vi "json_object.vi"(5 "text":string, 7 "ch":string, 9 "at":i32, 11 "error in (no error)":errorcluster) -> (4 "object":variant, 6 "text dup":string, 8 "ch out":string, 10 "at out":i32, 15 "error out":errorcluster)   [LabVIEW 2011]
doc: "Recursively return a JSON object (anything wrapped with {})."
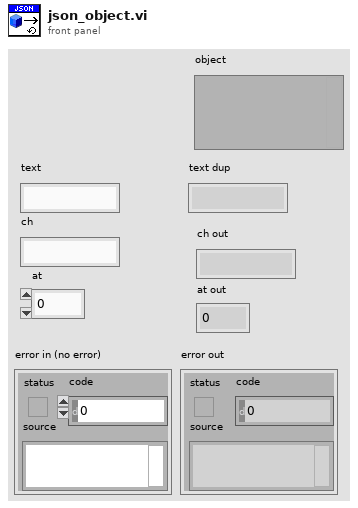
[diagram p1: front panel]
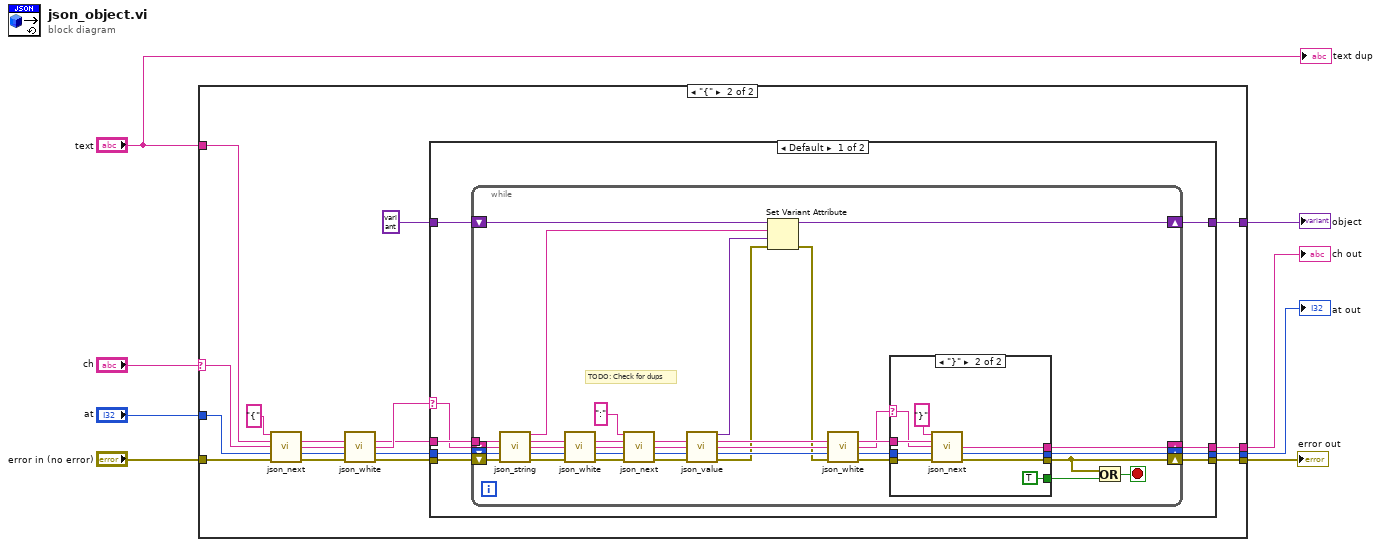
[diagram p0: block diagram]
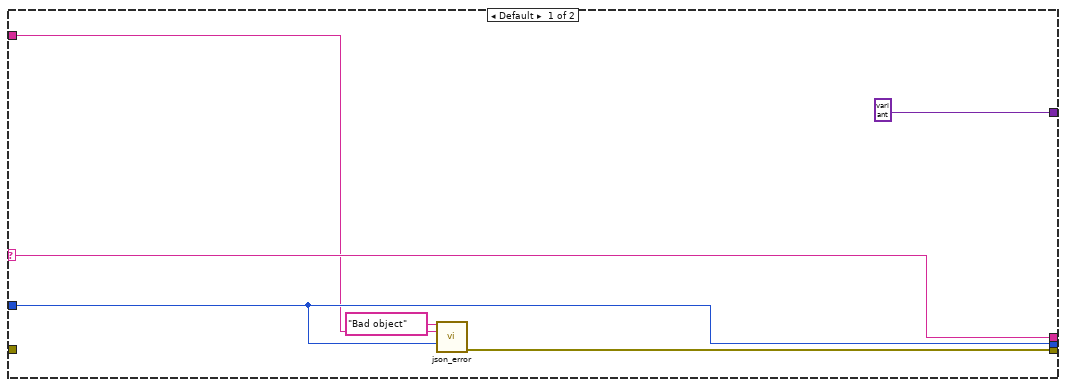
[diagram p2: hidden frame]
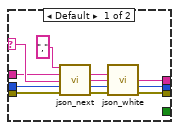
[diagram p3: hidden frame]
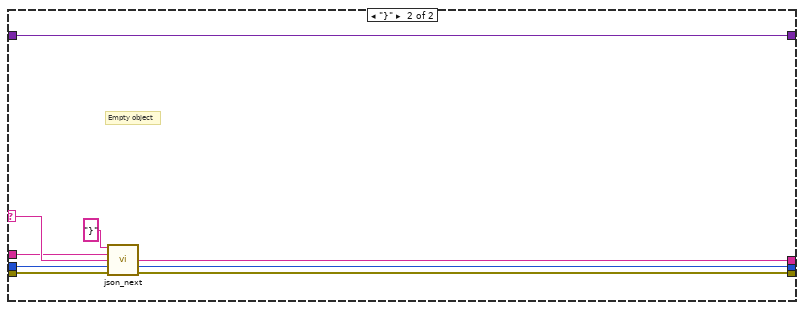
[diagram p4: hidden frame]
diagram:
  n1 = case shown="\"{\"" "ch" {
    selector: "ch" -> [w12 w31]
    tunnel: "error in (no error)" -> [_ w32]
    tunnel: "text" -> [w11 w29]
    tunnel: "at" -> [w13 w28]
    tunnel: [variant ("object") w21] -> w4
    tunnel: [w9 w20] -> w3
    tunnel: [w13 w16] -> w2
    tunnel: [w12 w15] -> w1
    frame Default {
      n2 = call "json_error.vi"("m"="Bad object", "text"=w11, "at"=w13) -> ("error out"=w9:errorcluster)  [unwired: 12 in]
    }
    frame "{" {
      n3 = call "json_next.vi"("c"="{", "text"=w29, "ch"=w31, "at"=w28, "error in (no error)"=w32) -> ("text dup"=w26:string, "ch out"=w25:string, "at out"=w24:i32, "error out"=w27:errorcluster)  [unwired: 7 in]
      n4 = call "json_white.vi"("text"=w26, "ch"=w25, "at"=w24, "error in (no error)"=w27) -> ("text dup"=w19:string, "ch out"=w22:string, "at out"=w18:i32, "error out"=w23:errorcluster)  [unwired: 8 in]
      n5 = case shown="Default" w22 {
        selector: w22 -> [w39 w101]
        tunnel: w23 -> [w41 w105]
        tunnel: [w36 w106] -> w21
        tunnel: [w35 w104] -> w20
        tunnel: w19 -> [w40 w99]
        tunnel: w18 -> [w38 w100]
        tunnel: variant ("object") -> [w37 w106]
        tunnel: [w34 w103] -> w16
        tunnel: [w33 w102] -> w15
        frame Default {
          n6 = while {
            tunnel: w40 -> [w75]
            shift-right: [w47] -> w33
            shift-left: w39 -> [w74]
            shift-right: [w48] -> w34
            shift-left: w38 -> [w73]
            shift-right: [w49] -> w36
            shift-left: w37 -> [w72]
            shift-right: [w44] -> w35
            shift-left: w41 -> [w76]
            stop <- w43 stop-if-true
            # "TODO: Check for dups"
            n7 = call "json_string.vi"("text"=w75, "ch"=w74, "at"=w73, "error in (no error)"=w76) -> ("string"=w71:string, "text dup"=w67:string, "ch out"=w68:string, "at"=w69:i32, "error out"=w70:errorcluster)  [unwired: 7 in]
            n8 = call "json_white.vi"("text"=w67, "ch"=w68, "at"=w69, "error in (no error)"=w70) -> ("text dup"=w63:string, "ch out"=w64:string, "at out"=w65:i32, "error out"=w66:errorcluster)  [unwired: 8 in]
            n9 = call "json_next.vi"("c"=":", "text"=w63, "ch"=w64, "at"=w65, "error in (no error)"=w66) -> ("text dup"=w58:string, "ch out"=w59:string, "at out"=w60:i32, "error out"=w61:errorcluster)  [unwired: 7 in]
            n10 = call "json_value.vi"("text"=w58, "ch"=w59, "at"=w60, "error in (no error)"=w61) -> ("value"=w57:variant, "text dup"=w54:string, "ch out"=w55:string, "at out"=w56:i32, "error out"=w46:errorcluster)  [unwired: 7 in]
            n11 = Set Variant Attribute(Variant=w72, name=w71, value=w57, error in=w46) -> (Variant out=w49:variant, error out=w45:errorcluster)  [unwired: 1 out]
            n12 = call "json_white.vi"("text"=w54, "ch"=w55, "at"=w56, "error in (no error)"=w45) -> ("text dup"=w51:string, "ch out"=w50:string, "at out"=w52:i32, "error out"=w53:errorcluster)  [unwired: 8 in]
            n13 = case shown="\"}\"" w50 {
              selector: w50 -> [w87 w94]
              tunnel: w53 -> [w88 w97]
              tunnel: w52 -> [w86 w95]
              tunnel: w51 -> [w85 w96]
              tunnel: [_ TRUE] -> w42
              tunnel: [w82 w91] -> w44
              tunnel: [w78 w90] -> w48
              tunnel: [w77 w89] -> w47
              frame Default {
                n14 = call "json_next.vi"("c"=",", "text"=w85, "ch"=w87, "at"=w86, "error in (no error)"=w88) -> ("text dup"=w79:string, "ch out"=w80:string, "at out"=w81:i32, "error out"=w83:errorcluster)  [unwired: 7 in]
                n15 = call "json_white.vi"("text"=w79, "ch"=w80, "at"=w81, "error in (no error)"=w83) -> ("ch out"=w77:string, "at out"=w78:i32, "error out"=w82:errorcluster)  [unwired: 8 in, 1 out]
              }
              frame "}" {
                n16 = call "json_next.vi"("c"="}", "text"=w96, "ch"=w94, "at"=w95, "error in (no error)"=w97) -> ("ch out"=w89:string, "at out"=w90:i32, "error out"=w91:errorcluster)  [unwired: 7 in, 1 out]
              }
            }
            n17 = Or(x=w44, y=w42) -> (x .or. y?=w43:bool)
          }
        }
        frame "}" {
          # "Empty object"
          n18 = call "json_next.vi"("c"="}", "text"=w99, "ch"=w101, "at"=w100, "error in (no error)"=w105) -> ("ch out"=w102:string, "at out"=w103:i32, "error out"=w104:errorcluster)  [unwired: 7 in, 1 out]
        }
      }
    }
  }
  "error out" <- w3
  "object" <- w4
  "ch out" <- w1
  "at out" <- w2
  "text dup" <- "text"
